vi "FixBundleNodes.vi"(8 "error in (no error)":errorcluster, 10 "Type":T1, 11 "VI Refnum":refnum<vi>) -> (0 "error out":errorcluster, 3 "VI Refnum":refnum<vi>)   [LabVIEW 2019, in "BlueSerializationScripts.lvlib"]
uses:
  BlueSerializationScripts.lvlib
  AccessDirection.ctl
  <vilib>/Utility/traverseref.llb/TRef TravTarget.ctl
  BlueSerialProviderGlobal.vi
  NI_Branches/BlueBranch_CLSUIP.lvlib
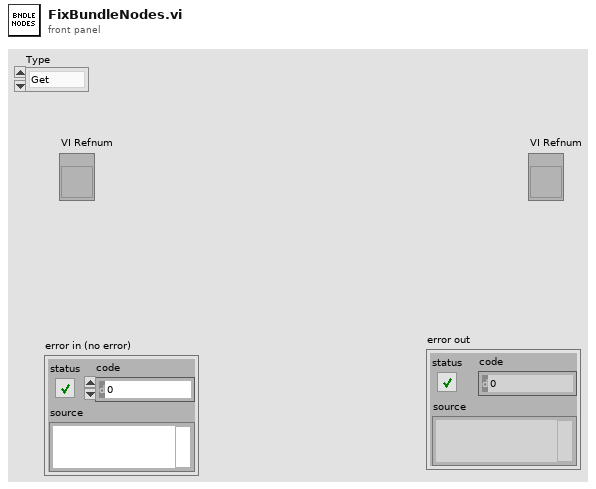
[diagram p1: front panel]
types:
  T1 = typedef "BlueSerializationScripts.lvlib/AccessDirection.ctl" = enum16{"Get", "Set"}
  T2 = typedef "TRef TravTarget.ctl" = enum16{"FP", "BD", "Other"}
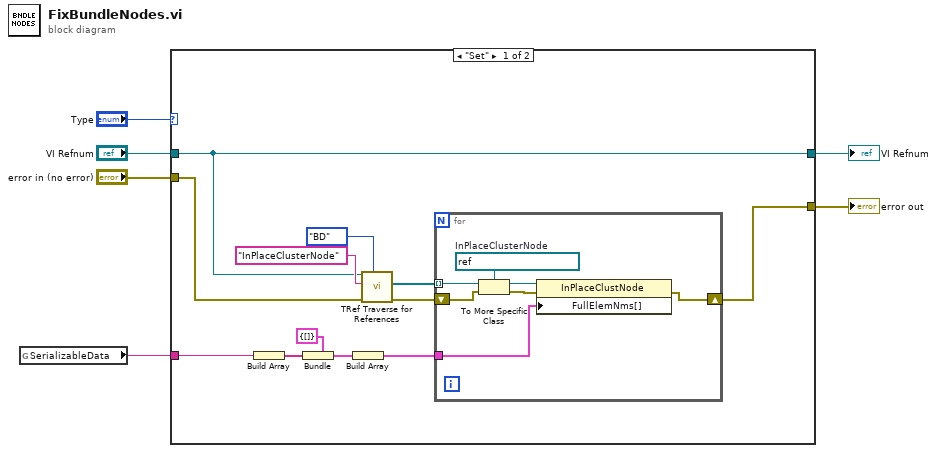
[diagram p0: block diagram]
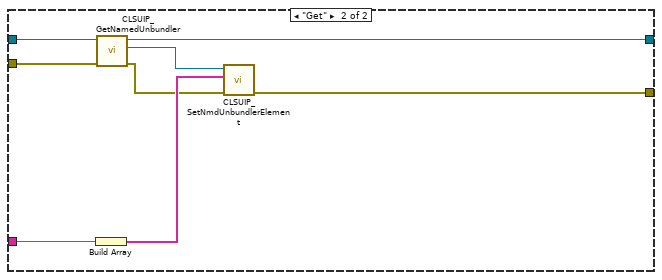
[diagram p2: hidden frame]
diagram:
  n1 = global read "BlueSerialProviderGlobal.vi" "SerializableData"() -> (w1:string)
  n2 = case shown="\"Set\"" "Type" {
    tunnel: "VI Refnum" -> [w16 w33]
    tunnel: [w16 w31] -> w5
    tunnel: "error in (no error)" -> [w10 w30]
    tunnel: [w8 w26] -> w3
    tunnel: w1 -> [w7 w29]
    frame "Set" {
      n3 = Build Array(w7) -> (w14:string[])
      n4 = Bundle(cluster=cluster{string[]} {[]}, w14) -> (w12:cluster{string[]})
      n5 = Build Array(w12) -> (w11:cluster{string[]}[])
      n6 = call <vilib>:"TRef Traverse for References.vi"("Traverse Target"=TRef_TravTarget."BD", "error in (no error)"=w10, "Class Name"="InPlaceClusterNode" ("y"), "VI Refnum"=w16) -> ("error out"=w9:errorcluster, "References"=w15:refnum<vi>[])  [unwired: 1 in, 5 out]
      n7 = for {
        tunnel: w15 -> [w25] mode=indexing
        tunnel: w11 -> [w22]
        shift-right: [w19] -> w8
        shift-left: w9 -> [w21]
        w24 = refnum<vi> refnum  # InPlaceClusterNode
        n8 = To More Specific Class(target class=w24, reference=w25, error in=w21) -> (specific class reference=w23:refnum<vi>, error out=w20:errorcluster)
        n9 = property class="InPlaceClustNode"(reference=w23, error in=w20, "FullElemNms[]"=w22) -> (error out=w19:errorcluster)  [unwired: 1 out]
      }
    }
    frame "Get" {
      n10 = Build Array(w29) -> (w32:string[])
      n11 = call "CLSUIP_GetNamedUnbundler.vi"("error in (no error)"=w30, "VI Refnum"=w33) -> ("error out"=w27:errorcluster, "NmdBundler Ref"=w28:refnum<vi>, "VI Refnum out"=w31:refnum<vi>)  [unwired: 7 in]
      n12 = call "CLSUIP_SetNmdUnbundlerElement.vi"("error in (no error)"=w27, "Element Names"=w32, "NmdUnbundler Ref"=w28) -> ("error out"=w26:errorcluster)  [unwired: 8 out]
    }
  }
  "VI Refnum" <- w5
  "error out" <- w3
